vi "HooksExtendPartial.vi"(8 "CurrentCount":i32, 9 "DesiredCount":i32) -> (2 "Done?":bool)   [LabVIEW 2013]
uses:
  Robot Global Data.vi
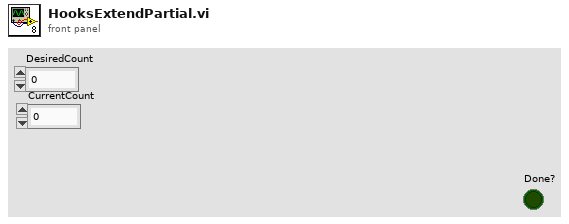
[diagram p1: front panel]
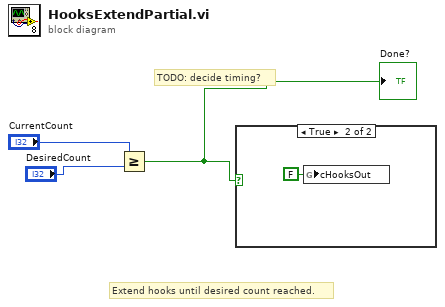
[diagram p0: block diagram]
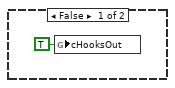
[diagram p2: hidden frame]
diagram:
  # "Extend hooks until desired count reached."
  # "TODO: decide timing?"
  n1 = Greater Or Equal?(x="CurrentCount", y="DesiredCount") -> (x >= y?=w1:bool)
  "Done?" <- w1
  n2 = case shown="True" w1 {
    frame False {
      n3 = global write "Robot Global Data.vi" "cHooksOut"(TRUE ("cHooksOut")) -> ()
    }
    frame True {
      n4 = global write "Robot Global Data.vi" "cHooksOut"(FALSE ("cHooksOut")) -> ()
    }
  }
